vi "FTW-Actor-GetInstanceConfiguration.vi"(0 "FTW Actor Instance":refnum<class "FTW-Actor-Instance.lvclass">, 11 "error in":errorcluster) -> (4 "FTW Actor Instance out":refnum<class "FTW-Actor-Instance.lvclass">, 6 "Identity":string, 15 "error out":errorcluster)   [LabVIEW 2013, in "FTW-Actor-Instance.lvclass"]
uses:
  FTW-Actor-Instance.lvclass
  FTW-Actor-Instance.lvclass/FTW-Actor-Instance.ctl
panel:
  # "Inputs"
  # "Outputs"
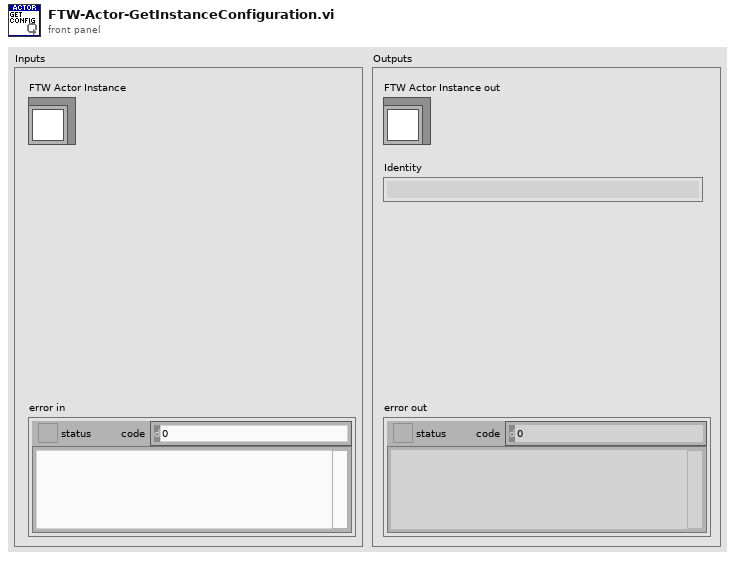
[diagram p1: front panel]
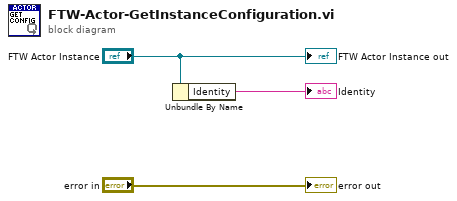
[diagram p0: block diagram]
diagram:
  n1 = Unbundle By Name("FTW Actor Instance") -> ("Identity"=→"Identity":string)
  "FTW Actor Instance out" <- "FTW Actor Instance"
  "error out" <- "error in"
